vi "rotate_3D_object.vi"(10 "Z (Pitch)":dbl, 11 "X (Roll)":dbl) -> (3 "3D Picture":refnum<vi>(3d-picture))   [LabVIEW 2017]
uses:
  <vilib>/picture/3D Picture Control/Object/Create Object (drawable).vi
  <vilib>/picture/3D Picture Control/Object/Add Object (no reference).vi
  <vilib>/picture/3D Picture Control/Object/Add Object (reference).vi
  <vilib>/picture/3D Picture Control/NI_3D Picture Control.lvlib
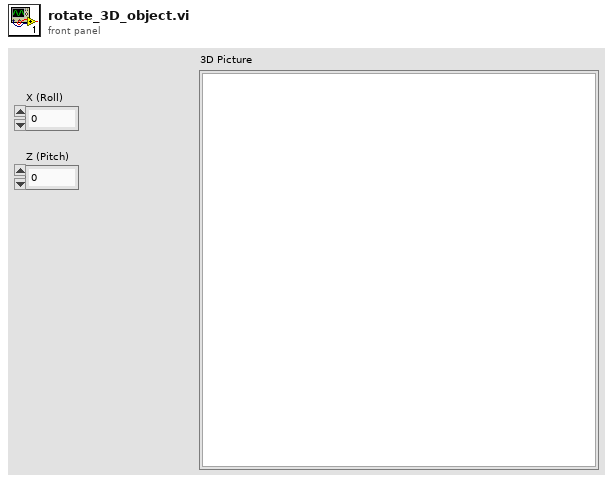
[diagram p1: front panel]
types:
  T1 = cluster{"element":sgl, "element 2":sgl, "element 3":sgl}
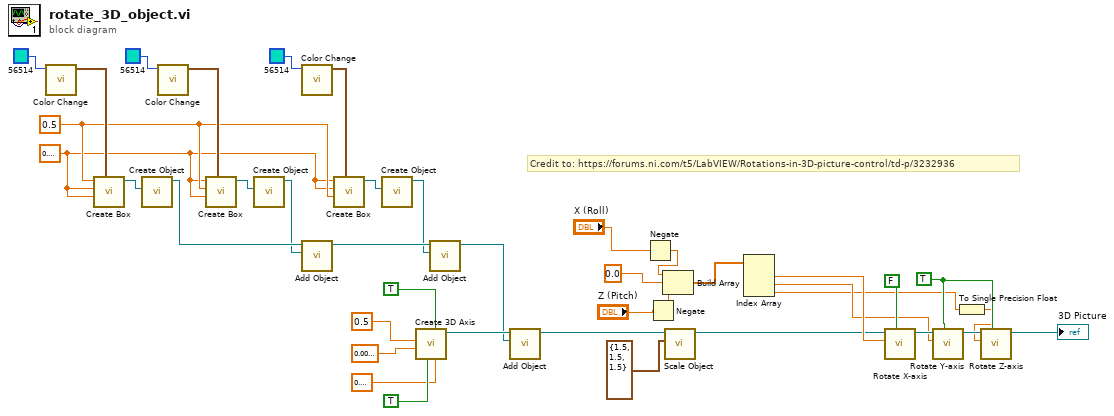
[diagram p0: block diagram]
diagram:
  w14 = TRUE ("Relative?")
  w19 = sgl 0.1 ("Character Size")
  w23 = sgl 0.5 ("Length")
  # "Credit to: https://forums.ni.com/t5/LabVIEW/Rotations-in-3D-picture-control/td-p/3232936"
  n1 = call <vilib>:"Color Change.vi"("Color"=u32 56514) -> ("RGBA"=w32:cluster{"R":sgl, "G":sgl, "B":sgl, "A":sgl})  [unwired: 10 in]
  n2 = call <vilib>:"Create Box.vi"("Color"=w32, "Length Z"=w19, "Length Y"=w19, "Length X"=w23) -> ("New Box Refnum"=w34:refnum<vi>)  [unwired: 6 in, 1 out]
  n3 = call-poly <vilib>:"Create Object.vi"("Geometry"=w34) -> ("Scene:New Object"=w28:refnum<vi>)  [unwired: 9 in, 1 out]
  n4 = call <vilib>:"Color Change.vi"("Color"=u32 56514) -> ("RGBA"=w29:cluster{"R":sgl, "G":sgl, "B":sgl, "A":sgl})  [unwired: 10 in]
  n5 = call <vilib>:"Create Box.vi"("Color"=w29, "Length Z"=w19, "Length Y"=w23, "Length X"=w19) -> ("New Box Refnum"=w31:refnum<vi>)  [unwired: 6 in, 1 out]
  n6 = call-poly <vilib>:"Create Object.vi"("Geometry"=w31) -> ("Scene:New Object"=w27:refnum<vi>)  [unwired: 9 in, 1 out]
  n7 = call <vilib>:"Color Change.vi"("Color"=u32 56514) -> ("RGBA"=w24:cluster{"R":sgl, "G":sgl, "B":sgl, "A":sgl})  [unwired: 10 in]
  n8 = call-poly <vilib>:"Add Object.vi"("New Object In"=w27, "Scene Object In"=w28) -> ("Scene Object Out"=w22:refnum<vi>)  [unwired: 8 in, 1 out]
  n9 = call <vilib>:"Create Box.vi"("Color"=w24, "Length Z"=w23, "Length Y"=w19, "Length X"=w19) -> ("New Box Refnum"=w26:refnum<vi>)  [unwired: 6 in, 1 out]
  n10 = call-poly <vilib>:"Create Object.vi"("Geometry"=w26) -> ("Scene:New Object"=w21:refnum<vi>)  [unwired: 9 in, 1 out]
  n11 = call <vilib>:"Create 3D Axis.vi"("Character Size"=sgl 0.1, "Half plane?"=TRUE, "Axis label?"=TRUE, "Radius"=sgl 0.01, "Length"=sgl 0.5) -> ("New Object Refnum"=w35:refnum<vi>)  [unwired: 5 in, 1 out]
  n12 = call-poly <vilib>:"Add Object.vi"("New Object In"=w21, "Scene Object In"=w22) -> ("Scene Object Out"=w20:refnum<vi>)  [unwired: 8 in, 1 out]
  n13 = call-poly <vilib>:"Add Object.vi"("New Object In"=w20, "Scene Object In"=w35) -> ("Scene Object Out"=w9:refnum<vi>)  [unwired: 7 in, 2 out]
  n14 = Negate(x="X (Roll)") -> (-x=w5:dbl)
  n15 = Negate(x="Z (Pitch)") -> (-x=w3:dbl)
  n16 = Build Array(w5, 0.0 ("element"), w3) -> (w12:dbl[])
  n17 = call <vilib>:"Scale Object.vi"("Scale"=T1 {"element"=1.5, "element 2"=1.5, "element 3"=1.5}, "Scene.Object In"=w9) -> ("Scene.Object Out"=w8:refnum<vi>)  [unwired: 8 in, 1 out]
  n18 = Index Array(array=w12) -> (element #1=w15:dbl, element #2=w13:dbl, element #3=w1:dbl)  [unwired: 3 in]
  n19 = call <vilib>:"Rotate X-axis.vi"("Relative?"=FALSE, "angle"=w15, "Scene Object In"=w8) -> ("Scene Object Out"=w18:refnum<vi>)  [unwired: 7 in, 1 out]
  n20 = call <vilib>:"Rotate Y-axis.vi"("Relative?"=w14, "angle"=w13, "Scene Object In"=w18) -> ("Scene Object Out"=w17:refnum<vi>)  [unwired: 7 in, 1 out]
  n21 = To Single Precision Float(number=w1) -> (single precision float=w2:sgl)
  n22 = call <vilib>:"Rotate Z-axis.vi"("Relative?"=w14, "angle"=w2, "Scene Object In"=w17) -> ("Scene Object Out"=→"3D Picture":refnum<vi>)  [unwired: 7 in, 1 out]
